vi "Configure Sequencer List Level.vi"(7 "Level (-30.0)":dbl=-30.0 format="%^.3e", 8 "error in (no error)":errorcluster, 9 "Index (0)":i32, 10 "Instance (1)":i32=1, 11 "VISA resource name":refnum<visa-resource-name>) -> (0 "error out":errorcluster, 3 "VISA resource name out":refnum<visa-resource-name>)   [LabVIEW 2015, in "Rohde&Schwarz CMXP GPRF.lvlib"]
doc: "Defines the level for the sequencer list entry with the selected Index.\n\nAttribute:\nRSCMXPGPRF_ATTR_SEQUENCER_LIST_LEVEL\n\nRemote-control command:\nSOURce:GPRF:GEN<i>:SEQuencer:LIST:LRMS"
uses:
  <instrlib>/Rohde&Schwarz CMXP GPRF/Rohde&Schwarz CMXP GPRF.lvlib
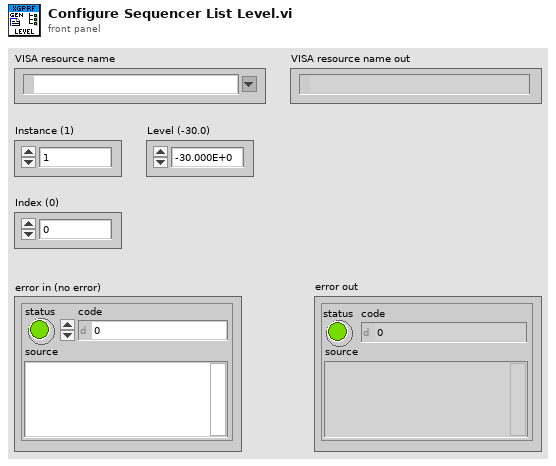
[diagram p1: front panel]
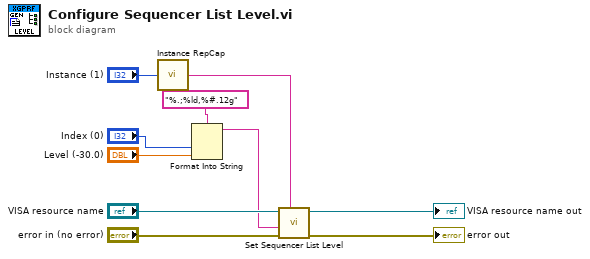
[diagram p0: block diagram]
diagram:
  n1 = call <instrlib>:"Instance RepCap.vi"("Instance in"="Instance (1)") -> ("Instance out"=w5:string)
  n2 = Format Into String(format string="%.;%ld,%#.12g", "Index (0)", "Level (-30.0)") -> (resulting string=w1:string)  [unwired: 2 in, 1 out]
  n3 = call "Set Sequencer List Level"("Repeated Capabilities"=w5, "error in (no error)"="error in (no error)", "Sequencer List Level ()"=w1, "instrument handle"="VISA resource name") -> ("error out"=→"error out":errorcluster, "instrument handle out"=→"VISA resource name out":refnum<visa-resource-name>)  [unwired: 6 in]
